vi "SPlowClamp.vi"(13 "SP":dbl) -> (2 "clampedSP":dbl)   [LabVIEW 2016]
doc: "For setpoints <=2%, the Aalborg shuts, and performs self-zeroing- so for calculations, SPs of 2 or below should be treated as zero"
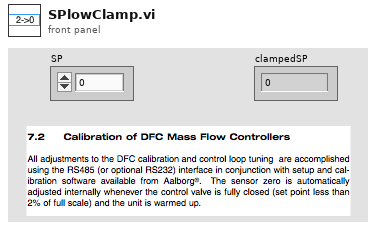
[diagram p1: front panel]
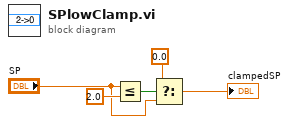
[diagram p0: block diagram]
diagram:
  n1 = Less Or Equal?(x="SP", y=2.0) -> (x <= y?=w3:bool)
  n2 = Select(t=0.0, s=w3, f="SP") -> (s? t:f=→"clampedSP":dbl)
